vi "test Multiple Request Response.vi"(8 "error in (no error)":errorcluster, 11 "TestCase in":refnum<class "Single Consumer Test Case.lvclass">) -> (0 "error out":errorcluster, 3 "TestCase out":refnum<class "Single Consumer Test Case.lvclass">)   [LabVIEW 2027, in "Single Consumer Test Case.lvclass"]
uses:
  Single Consumer Test Case.lvclass
  Support/Messages/Consumer Name Request Message/Consumer Name Request Message.lvclass
  C:/NetCore/niveristand-custom-device-message-library/Source/Message/Abstract Request Message/Abstract Request Message.lvclass
  Message/Shutdown Message/Shutdown Message.lvclass
  Support/Message List Action.ctl
  Support/Messages/Test Message/Test Message.lvclass
  Single Consumer Test Case.lvclass/Single Consumer Test Case.ctl
  Message/Abstract Request Message/Abstract Request Message.lvclass
  C:/NetCore/niveristand-custom-device-message-library/Source/Message/Abstract Message/Abstract Message.lvclass
  Producer/Abstract Producer/Abstract Producer.lvclass
  C:/Program Files/National Instruments/LabVIEW 2027/vi.lib/addons/_JKI Toolkits/VI Tester/TestCase.llb/TestCase.lvclass
  <vilib>/addons/_JKI Toolkits/VI Tester/TestCase.llb/TestCase.lvclass
  Consumer/Abstract Consumer/Abstract Consumer.lvclass
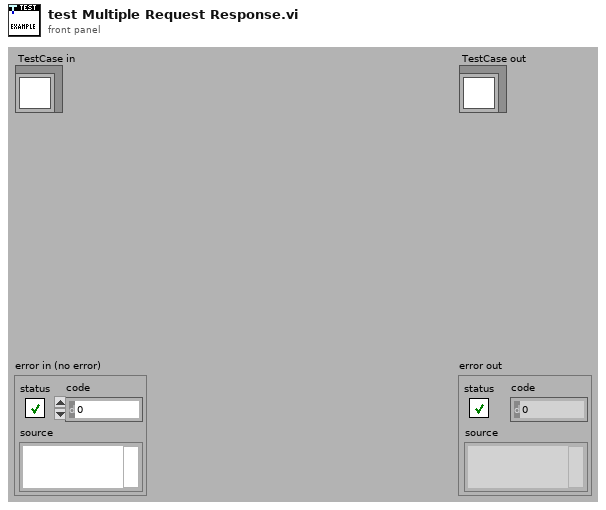
[diagram p1: front panel]
types:
  T1 = typedef "Message List Action.ctl" = enum16{"Get", "Add", "Reset"}
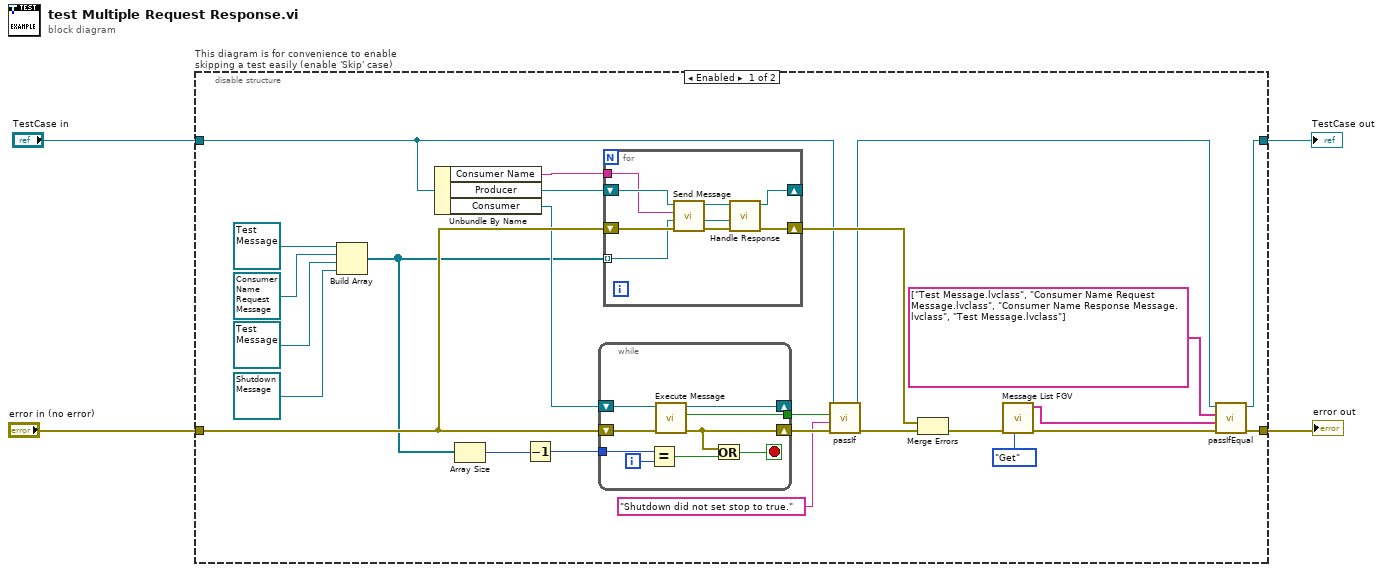
[diagram p0: block diagram]
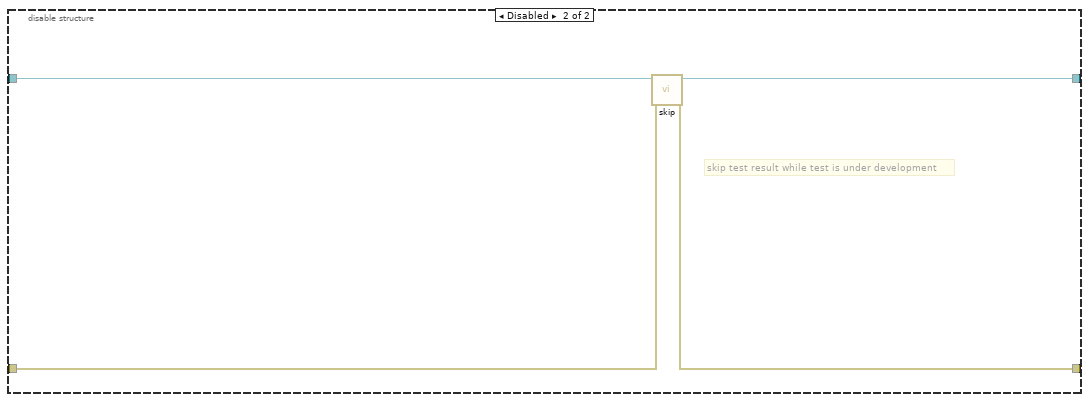
[diagram p2: hidden frame]
diagram:
  n1 = disable-structure "This diagram is for convenience to enable skipping a test easily (enable 'Skip' case)" shown="Enabled" {
    disable-tunnel: "TestCase in" -> [w17 w51]
    disable-tunnel: [w9 w49] -> w1
    disable-tunnel: [w11 w50] -> w3
    disable-tunnel: "error in (no error)" -> [w29 w48]
    frame Enabled {
      n2 = Build Array(refnum<class "Test Message.lvclass"> refnum ("Test Message.lvclass"), refnum<class "Consumer Name Request Message.lvclass"> refnum ("Consumer Name Request Message.lvclass"), refnum<class "Test Message.lvclass"> refnum ("Test Message.lvclass"), refnum<class "Shutdown Message.lvclass"> refnum ("Messaging.lvlib:Message.lvlib:Shutdown Message.lvclass")) -> (w20:refnum<class "Abstract Request Message.lvclass">[])
      n3 = Unbundle By Name(w17) -> ("Consumer Name"=w26:string, "Producer"=w27:refnum<class "Abstract Producer.lvclass">, "Consumer"=w28:refnum<class "Abstract Consumer.lvclass">)
      n4 = Array Size(array=w20) -> (size(s)=w19:i32)
      n5 = Decrement(x=w19) -> (x-1=w14:i32)
      n6 = while {
        shift-right: [w36] -> w23
        shift-left: w29 -> [w38]
        shift-right: [w34] -> _
        shift-left: w28 -> [w35]
        tunnel: w14 -> [w33]
        tunnel: [w30] -> w16
        i -> [w32]
        stop <- w37 stop-if-true
        n7 = Equal?(x=w33, y=w32) -> (x = y?=w31:bool)
        n8 = call "Execute Message.vi"("error in (no error)"=w38, "Abstract Consumer in"=w35) -> ("error out"=w36:errorcluster, "Stop?"=w30:bool, "Abstract Consumer out"=w34:refnum<class "Abstract Consumer.lvclass">)  [unwired: 6 in, 1 out]
        n9 = Or(x=w36, y=w31) -> (x .or. y?=w37:bool)
      }
      n10 = for {
        shift-right: [w40] -> w22
        shift-left: w29 -> [w47]
        shift-right: [w39] -> _
        shift-left: w27 -> [w46]
        tunnel: w26 -> [w45]
        tunnel: w20 -> [w44] mode=indexing
        n11 = call-dynamic "Send Message.vi"("error in (no error)"=w47, "Message in"=w44, "Consumer in"=w45, "Abstract Producer in"=w46) -> ("error out"=w43:errorcluster, "Message out"=w41:refnum<class "Abstract Message.lvclass">, "Abstract Producer out"=w42:refnum<class "Abstract Producer.lvclass">)  [unwired: 4 in, 1 out]
        n12 = call-dynamic "Handle Response.vi"("error in (no error)"=w43, "Abstract Response Message"=w41, "Abstract Producer in"=w42) -> ("error out"=w40:errorcluster, "Abstract Producer out"=w39:refnum<class "Abstract Producer.lvclass">)  [unwired: 7 in]
      }
      n13 = call-dynamic "passIf.vi"("error in (no error)"=w23, "message (\"\")"="Shutdown did not set stop to true." ("message (\"\")"), "pass"=w16, "TestCase in"=w17) -> ("error out"=w18:errorcluster, "TestCase out"=w10:refnum<class "Single Consumer Test Case.lvclass">)  [unwired: 6 in]
      n14 = Merge Errors(w22, w18) -> (w21:errorcluster)
      n15 = call "Message List FGV.vi"("Action (Get)"=Message_List_Action."Get", "error in (no error)"=w21) -> ("error out"=w12:errorcluster, "Messages"=w8:string[])  [unwired: 8 in]
      n16 = call-dynamic "passIfEqual.vi"("error in (no error)"=w12, "y"=w8, "x"=string[] ["Test Message.lvclass", "Consumer Name Request Message.lvclass", "Consumer Name Response Message.lvclass", "Test Message.lvclass"], "TestCase in"=w10) -> ("error out"=w11:errorcluster, "TestCase out"=w9:refnum<class "Single Consumer Test Case.lvclass">)  [unwired: 6 in]
    }
    frame Disabled {
      # "skip test result while test is under development"
      n17 = call <vilib>:"skip.vi"("error in (no error)"=w48, "TestCase in"=w51) -> ("error out"=w50:errorcluster, "TestCase out"=w49:refnum<class "Single Consumer Test Case.lvclass">)  [unwired: 8 in]
    }
  }
  "error out" <- w3
  "TestCase out" <- w1
